vi "UI_updateBoolCtrlEnabled.vi"(8 "error in (no error)":errorcluster, 10 "Enabled?":bool, 11 "boolRef":refnum<vi>) -> (0 "error out":errorcluster)   [LabVIEW 2020]
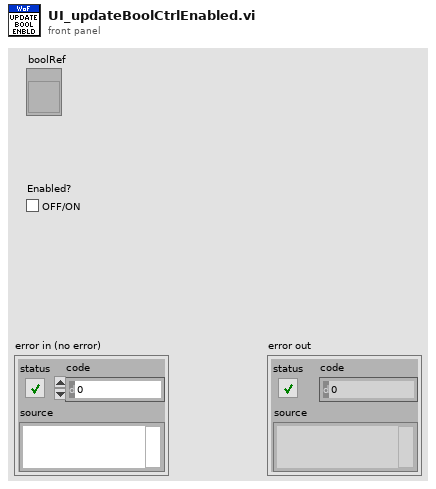
[diagram p1: front panel]
types:
  T1 = enum8{"Enabled", "Disabled", "Disabled and Grayed Out"}
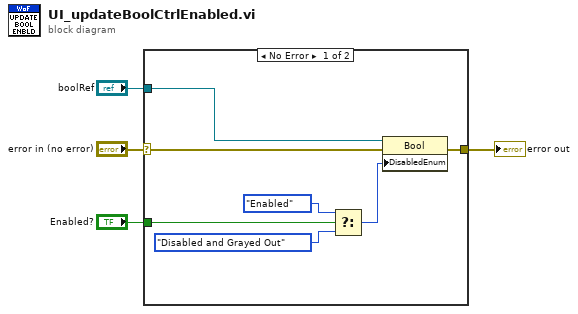
[diagram p0: block diagram]
diagram:
  n1 = case shown="No Error" "error in (no error)" {
    selector: "error in (no error)" -> [w11 w12]
    tunnel: "boolRef" -> [w10 _]
    tunnel: "Enabled?" -> [w8 _]
    tunnel: [w5 w12] -> w1
    frame No Error {
      n2 = Select(t=T1."Enabled" ("Disabled"), s=w8, f=T1."Disabled and Grayed Out" ("Disabled")) -> (s? t:f=w6:T1)
      n3 = property class="Bool"(reference=w10, error in=w11, "DisabledEnum"=w6) -> (error out=w5:errorcluster)  [unwired: 1 out]
    }
    frame Error {
    }
  }
  "error out" <- w1
